vi "Create_Trajectory_Read_Field_Pic.vi"(11 "file name":string) -> (0 "error out":errorcluster, 1 "error out 2":errorcluster, 2 "image data":T1, 3 "Refnum out":T2)   [LabVIEW 2019]
uses:
  <vilib>/vision/Image Controls.llb/IMAQ Image.ctl
  <vilib>/picture/picture.llb/imagedata.ctl
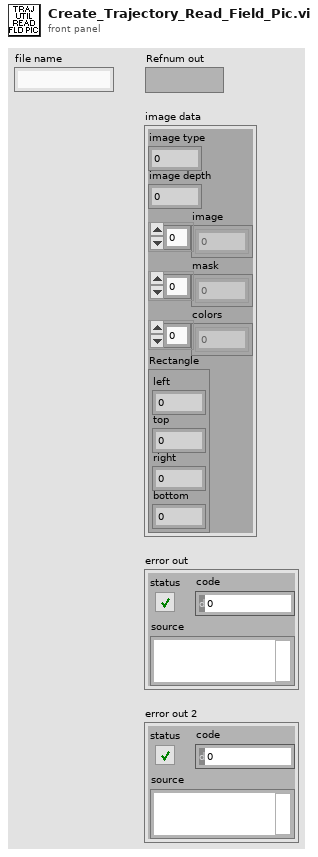
[diagram p1: front panel]
types:
  T1 = typedef "imagedata.ctl" = cluster{"image type":i32, "image depth":i32, "image":u8[], "mask":u8[], "colors":u32[], "Rectangle":cluster{"left":i16, "top":i16, "right":i16, "bottom":i16}}
  T2 = typedef "IMAQ Image.ctl" = refnum<image>
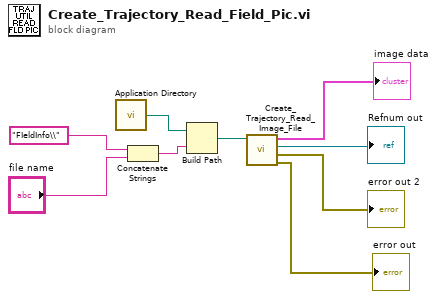
[diagram p0: block diagram]
diagram:
  n1 = call <vilib>:"Application Directory.vi"() -> ("Application Directory"=w2:path)
  n2 = Concatenate Strings("FIeldInfo\\" ("string"), "file name") -> (w9:string)
  n3 = Build Path(base path=w2, name or relative path=w9) -> (appended path=w3:path)
  n4 = call "Create_Trajectory_Read_Image_File.vi"("file"=w3) -> ("error out"=→"error out":errorcluster, "error out 2"=→"error out 2":errorcluster, "Image Out"=→"Refnum out":T2, "image data"=→"image data":T1)  [unwired: 7 in]
